vi "red_tweezers_globals_INTERNAL_VOLATILE.vi"() -> ()   [LabVIEW 2015]
panel:
  in  "Save Settings On Exit":bool
  in  "Camera Settings":cluster{"Gain":dbl, "Exposure":dbl, "Set":bool}
  in  "iPad Plug-in VI References (set by plugins_load.vi)":refnum<vi>[](array[refnum])
  in  "Current Camera VI":path
  out "Video Frame Rate":dbl(knob)=428.7584340568731 scale=0.0..1000.0 scale format="%.1f"
  out "Tracked Spot Positions (stereo)":T1(array[cluster])
  out "Tracked Spot Positions (3D)":cluster{"x":dbl, "y":dbl, "Z":dbl}[](array[cluster])
  in  "Current Settings File":path
  # "The controls here should NOT be saved when the program exits."
  # "current positions of the spots- you might want to use the queue instead, I think"
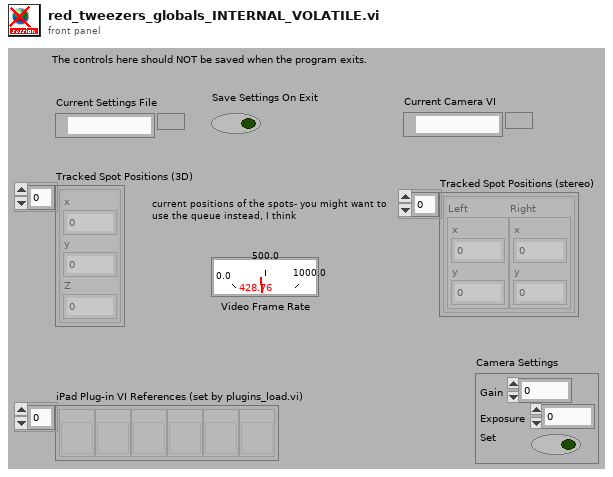
[diagram p1: front panel]
types:
  T1 = cluster{"Left":cluster{"x":dbl, "y":dbl}, "Right":cluster{"x":dbl, "y":dbl}}[]
diagram:
